vi "Check White Balance Changed Port.vi"(11 "Port White Balance":refnum<vi>) -> ()   [LabVIEW 2025]
uses:
  <vilib>/Rock Robotics/Network Tables/NT Read Number.vi
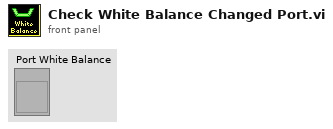
[diagram p1: front panel]
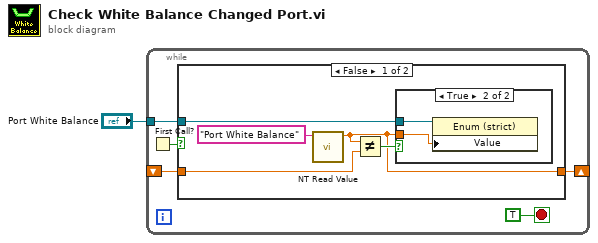
[diagram p0: block diagram]
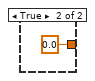
[diagram p3: hidden frame]
diagram:
  n1 = while {
    shift-right: [w5] -> _
    shift-left: _ -> [w4]
    tunnel: "Port White Balance" -> [w2]
    stop <- TRUE stop-if-true
    n2 = First Call?() -> (First Call?: T/F=w6:bool)
    n3 = case shown="False" w6 {
      tunnel: [w8 0.0 ("Numeric")] -> w5
      tunnel: w4 -> [w11 _]
      tunnel: w2 -> [w9 _]
      frame False {
        n4 = call-poly <vilib>:"NT Read Value.vi"("name"="Port White Balance" ("Name")) -> ("value"=w8:dbl)  [unwired: 8 in, 2 out]
        n5 = Not Equal?(x=w8, y=w11) -> (x != y?=w10:bool)
        n6 = case shown="True" w10 {
          tunnel: w9 -> [_ w13]
          tunnel: w8 -> [_ w12]
          frame False {
          }
          frame True {
            n7 = property class="Enum (strict)"(reference=w13, "Value"=w12) -> ()  [unwired: 1 in, 2 out]
          }
        }
      }
      frame True {
      }
    }
  }
